vi "Remove Item by name array.vi"(8 "error in (no error)":errorcluster, 10 "Name Array":string[](array[string]), 11 "JSON Value In":refnum<class "JSON Value.lvclass">) -> (0 "error out":errorcluster, 1 "removed":bool, 3 "JSON Value Out":refnum<class "JSON Value.lvclass">)   [LabVIEW 2011, in "JSON Value.lvclass"]
doc: "Removes a JSON Value in a JSON collection by it's path. The paths is an array of strings.\nThe first element is the top level name. For elements in an array you can use a %d formatted number to index an element out.\n\nCopyright 2012 James David Powell, Shaun Rumbell and Ton Plomp\nMore information on http://lavag.org/topic/16217-cr-json-labview"
uses:
  JSON Value.lvclass
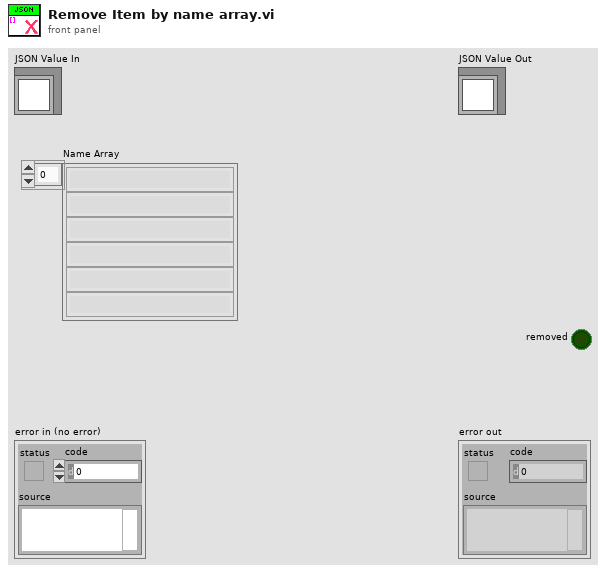
[diagram p1: front panel]
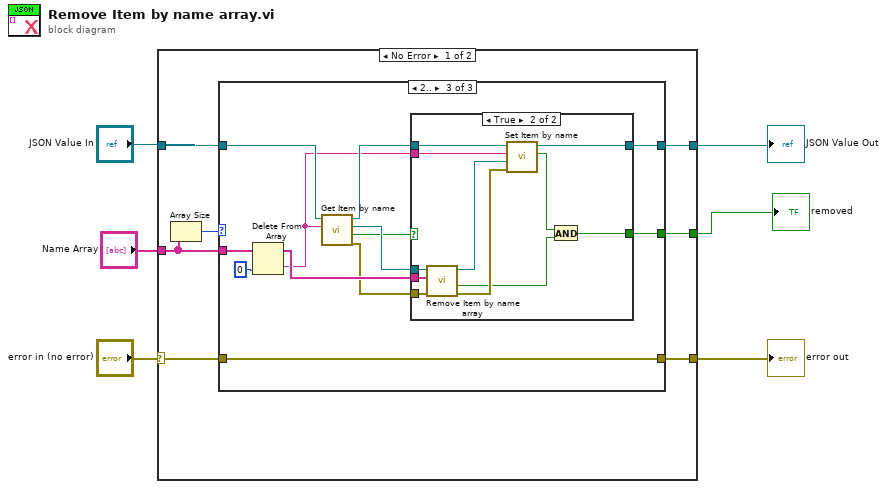
[diagram p0: block diagram]
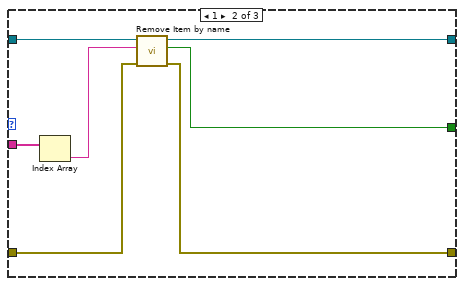
[diagram p3: hidden frame]
diagram:
  n1 = case shown="No Error" "error in (no error)" {
    selector: "error in (no error)" -> [w8 w47]
    tunnel: [w12 w48] -> w5
    tunnel: "JSON Value In" -> [w13 w48]
    tunnel: "Name Array" -> [w10 _]
    tunnel: [w11 _] -> w2
    tunnel: [w7 w47] -> w1
    frame No Error {
      n2 = Array Size(array=w10) -> (size(s)=w9:i32)
      n3 = case shown="2.." w9 {
        tunnel: w13 -> [w15 w22 w30]
        tunnel: [w15 w21 w26] -> w12
        tunnel: [_ w16 w29] -> w11
        tunnel: w10 -> [_ w20 w28]
        tunnel: w8 -> [w14 w18 w24]
        tunnel: [w14 w17 w24] -> w7
        frame 0, Default {
        }
        frame 1 {
          n4 = Index Array(array=w20) -> (element=w19:string)  [unwired: 1 in]
          n5 = call-dynamic "Remove Item by name.vi"("error in (no error)"=w18, "name"=w19, "JSON Value In"=w22) -> ("error out"=w17:errorcluster, "removed"=w16:bool, "JSON Value Out"=w21:refnum<class "JSON Value.lvclass">)  [unwired: 6 in]
        }
        frame 2.. {
          n6 = Delete From Array(array=w28, index=0) -> (deleted portion=w25:string, array with subset deleted=w32:string[])  [unwired: 1 in]
          n7 = call-dynamic "Get Item by name.vi"("name"=w25, "JSON Value In"=w30) -> ("error out"=w31:errorcluster, "found"=w23:bool, "Value"=w33:refnum<class "JSON Value.lvclass">, "JSON Value Out"=w27:refnum<class "JSON Value.lvclass">)  [unwired: 6 in]
          n8 = case shown="True" w23 {
            tunnel: w33 -> [_ w46]
            tunnel: w32 -> [_ w45]
            tunnel: w31 -> [_ w44]
            tunnel: [_ w36] -> w29
            tunnel: w27 -> [w35 w43]
            tunnel: [w35 w42] -> w26
            tunnel: w25 -> [_ w40]
            frame False {
            }
            frame True {
              n9 = call "Remove Item by name array.vi"("error in (no error)"=w44, "Name Array"=w45, "JSON Value In"=w46) -> ("error out"=w41:errorcluster, "removed"=w37:bool, "JSON Value Out"=w39:refnum<class "JSON Value.lvclass">)  [unwired: 6 in]
              n10 = call-dynamic "Set Item by name.vi"("error in (no error)"=w41, "Value"=w39, "name"=w40, "JSON Value In"=w43) -> ("replaced"=w38:bool, "JSON Value Out"=w42:refnum<class "JSON Value.lvclass">)  [unwired: 5 in, 1 out]
              n11 = And(x=w38, y=w37) -> (x .and. y?=w36:bool)
            }
          }
        }
      }
    }
    frame Error {
    }
  }
  "error out" <- w1
  "JSON Value Out" <- w5
  "removed" <- w2
